vi "main.vi"() -> ()   [LabVIEW 2023] (continued)
C4\r\n      3444  0CF102A7   00000004    8        30\t75\tE0\t2E\t80\tFF\tFF\tFD\r\n      3443  0C3C4D4A   00000004    8        BE\tFF\tFF\t7F\t18\tFF\tFF\t5A\r\n      3443  0CF101A7   00000004    8        68\t00\t97\tCC\t00\t19\t39\tC6\r\n      3442  18F120F0   00000004    8        2B\t75\t60\tB1\tB0\t01\tFF\tFF\r\n      3441  18F11FF0   00000004    8        FF\t3F\t90\t68\t88\t1B\t10\tAC\r\n      3432  1FFFFFFF   00000004    8        00\t00\tFF\tFF\tFF\tFF\tFF\tFF\r\n      3423  0CF102A7   00000004    8        30\t75\tE0\t2E\t80\tFF\tFF\tFD\r\n      3423  0CF101A7   00000004    8        68\t00\t97\tCC\t00\t19\t39\tC5\r\n      3422  1FFFFFFF   00000004    8        00\t00\tFF\tFF\tFF\tFF\tFF\tFF\r\n      3412  1FFFFFFF   00000004    8        00\t00\tFF\tFF\tFF\tFF\tFF\tFF\r\n      3403  0CF102A7   00000004    8        30\t75\tE0\t2E\t80\tFF\tFF\tFD\r\n      3444  0CF103A7   00000004    8        17\t1F\t08\t60\tB1\t1F\t08\t5A\r\n      3444  0CF102A7   00000004    8        30\t75\tE0\t2E\t80\tFF\tFF\tFD\r\n      3443  0C3C4D4A   00000004    8        BE\tFF\tFF\t7F\t18\tFF\tFF\t5A\r\n      3443  0CF101A7   00000004    8        68\t00\t97\tCC\t00\t19\t39\tC6\r\n      3442  18F120F0   00000004    8        2B\t75\t60\tB1\tB0\t01\tFF\tFF\r\n      3441  18F11FF0   00000004    8        FF\t3F\t90\t68\t88\t1B\t10\tAC\r\n      3432  1FFFFFFF   00000004    8        00\t00\tFF\tFF\tFF\tFF\tFF\tFF\r\n      3423  0CF102A7   00000004    8        30\t75\tE0\t2E\t80\tFF\tFF\tFD\r\n      3423  0CF101A7   00000004    8        68\t00\t97\tCC\t00\t19\t39\tC5\r\n      3422  1FFFFFFF   00000004    8        00\t00\tFF\tFF\tFF\tFF\tFF\tFF\r\n      3412  1FFFFFFF   00000004    8        00\t00\tFF\tFF\tFF\tFF\tFF\tFF\r\n      3445  0CF104A7   00000004    8        F0\t60\t22\tFC\tFF\tFF\tFF\t5A\r\n      3444  0CF103A7   00000004    8        17\t1F\t08\t60\tB1\t1F\t08\t5A\r\n      3444  0CF102A7   00000004    8        30\t75\tE0\t2E\t80\tFF\tFF\tFD\r\n      3443  0C3C4D4A   00000004    8        BE\tFF\tFF\t7F\t18\tFF\tFF\t5A\r\n      3443  0CF101A7   00000004    8        68\t00\t97\tCC\t00\t19\t39\tC6\r\n      3442  18F120F0   00000004    8        2B\t75\t60\tB1\tB0\t01\tFF\tFF\r\n      3441  18F11FF0   00000004    8        FF\t3F\t90\t68\t88\t1B\t10\tAC\r\n      3432  1FFFFFFF   00000004    8        00\t00\tFF\tFF\tFF\tFF\tFF\tFF\r\n      3423  0CF102A7   00000004    8        30\t75\tE0\t2E\t80\tFF\tFF\tFD\r\n      3423  0CF101A7   00000004    8        68\t00\t97\tCC\t00\t19\t39\tC5\r\n      3422  1FFFFFFF   00000004    8        00\t00\tFF\tFF\tFF\tFF\tFF\tFF\r\n      3445  18F106A7   00000004    8        00\tF7\tFF\tFF\tFF\tFF\tFF\tB5\r\n      3445  0CF104A7   00000004    8        F0\t60\t22\tFC\tFF\tFF\tFF\t5A\r\n      3444  0CF103A7   00000004    8        17\t1F\t08\t60\tB1\t1F\t08\t5A\r\n      3444  0CF102A7   00000004    8        30\t75\tE0\t2E\t80\tFF\tFF\tFD\r\n      3443  0C3C4D4A   00000004    8        BE\tFF\tFF\t7F\t18\tFF\tFF\t5A\r\n      3443  0CF101A7   00000004    8        68\t00\t97\tCC\t00\t19\t39\tC6\r\n      3442  18F120F0   00000004    8        2B\t75\t60\tB1\tB0\t01\tFF\tFF\r\n      3441  18F11FF0   00000004    8        FF\t3F\t90\t68\t88\t1B\t10\tAC\r\n      3432  1FFFFFFF   00000004    8        00\t00\tFF\tFF\tFF\tFF\tFF\tFF\r\n      3423  0CF102A7   00000004    8        30\t75\tE0\t2E\t80\tFF\tFF\tFD\r\n      3423  0CF101A7   00000004    8        68\t00\t97\tCC\t00\t19\t39\tC5\r\n      3446  18F121F0   00000004    8        09\t33\t00\t00\tFF\tFF\tB0\t01\r\n      3445  18F106A7   00000004    8        00\tF7\tFF\tFF\tFF\tFF\tFF\tB5\r\n      3445  0CF104A7   00000004    8        F0\t60\t22\tFC\tFF\tFF\tFF\t5A\r\n      3444  0CF103A7   00000004    8        17\t1F\t08\t60\tB1\t1F\t08\t5A\r\n      3444  0CF102A7   00000004    8        30\t75\tE0\t2E\t80\tFF\tFF\tFD\r\n      3443  0C3C4D4A   00000004    8        BE\tFF\tFF\t7F\t18\tFF\tFF\t5A\r\n      3443  0CF101A7   00000004    8        68\t00\t97\tCC\t00\t19\t39\tC6\r\n      3442  18F120F0   00000004    8        2B\t75\t60\tB1\tB0\t01\tFF\tFF\r\n      3441  18F11FF0   00000004    8        FF\t3F\t90\t68\t88\t1B\t10\tAC\r\n      3432  1FFFFFFF   00000004    8        00\t00\tFF\tFF\tFF\tFF\tFF\tFF\r\n      3423  0CF102A7   00000004    8        30\t75\tE0\t2E\t80\tFF\tFF\tFD\r\n      3447  1FFFFFFF   00000004    8        00\t00\tFF\tFF\tFF\tFF\tFF\tFF\r\n      3446  18F121F0   00000004    8        09\t33\t00\t00\tFF\tFF\tB0\t01\r\n      3445  18F106A7   00000004    8        00\tF7\tFF\tFF\tFF\tFF\tFF\tB5\r\n      3445  0CF104A7   00000004    8        F0\t60\t22\tFC\tFF\tFF\tFF\t5A\r\n      3444  0CF103A7   00000004    8        17\t1F\t08\t60\tB1\t1F\t08\t5A\r\n      3444  0CF102A7   00000004    8        30\t75\tE0\t2E\t80\tFF\tFF\tFD\r\n      3443  0C3C4D4A   00000004    8        BE\tFF\tFF\t7F\t18\tFF\tFF\t5A\r\n      3443  0CF101A7   00000004    8        68\t00\t97\tCC\t00\t19\t39\tC6\r\n      3442  18F120F0   00000004    8        2B\t75\t60\tB1\tB0\t01\tFF\tFF\r\n      3441  18F11FF0   00000004    8        FF\t3F\t90\t68\t88\t1B\t10\tAC\r\n      3432  1FFFFFFF   00000004    8        00\t00\tFF\tFF\tFF\tFF\tFF\tFF\r\n      3452  1FFFFFFF   00000004    8        00\t00\tFF\tFF\tFF\tFF\tFF\tFF\r\n      3447  1FFFFFFF   00000004    8        00\t00\tFF\tFF\tFF\tFF\tFF\tFF\r\n      3446  18F121F0   00000004    8        09\t33\t00\t00\tFF\tFF\tB0\t01\r\n      3445  18F106A7   00000004    8        00\tF7\tFF\tFF\tFF\tFF\tFF\tB5\r\n      3445  0CF104A7   00000004    8        F0\t60\t22\tFC\tFF\tFF\tFF\t5A\r\n      3444  0CF103A7   00000004    8        17\t1F\t08\t60\tB1\t1F\t08\t5A\r\n      3444  0CF102A7   00000004    8        30\t75\tE0\t2E\t80\tFF\tFF\tFD\r\n      3443  0C3C4D4A   00000004    8        BE\tFF\tFF\t7F\t18\tFF\tFF\t5A\r\n      3443  0CF101A7   00000004    8        68\t00\t97\tCC\t00\t19\t39\tC6\r\n      3442  18F120F0   00000004    8        2B\t75\t60\tB1\tB0\t01\tFF\tFF\r\n      3441  18F11FF0   00000004    8        FF\t3F\t90\t68\t88\t1B\t10\tAC\r\n      3462  1FFFFFFF   00000004    8        00\t20\tFF\tFF\tFF\tFF\tFF\tFF\r\n      3452  1FFFFFFF   00000004    8        00\t00\tFF\tFF\tFF\tFF\tFF\tFF\r\n      3447  1FFFFFFF   00000004    8        00\t00\tFF\tFF\tFF\tFF\tFF\tFF\r\n      3446  18F121F0   00000004    8        09\t33\t00\t00\tFF\tFF\tB0\t01\r\n      3445  18F106A7   00000004    8        00\tF7\tFF\tFF\tFF\tFF\tFF\tB5\r\n      3445  0CF104A7   00000004    8        F0\t60\t22\tFC\tFF\tFF\tFF\t5A\r\n      3444  0CF103A7   00000004    8        17\t1F\t08\t60\tB1\t1F\t08\t5A\r\n      3444  0CF102A7   00000004    8        30\t75\tE0\t2E\t80\tFF\tFF\tFD\r\n      3443  0C3C4D4A   00000004    8        BE\tFF\tFF\t7F\t18\tFF\tFF\t5A\r\n      3443  0CF101A7   00000004    8        68\t00\t97\tCC\t00\t19\t39\tC6\r\n      3442  18F120F0   00000004    8        2B\t75\t60\tB1\tB0\t01\tFF\tFF\r\n      3463  0CF101A7   00000004    8        68\t00\t97\tCC\t00\t19\t39\tC7\r\n      3462  1FFFFFFF   00000004    8        00\t20\tFF\tFF\tFF\tFF\tFF\tFF\r\n      3452  1FFFFFFF   00000004    8        00\t00\tFF\tFF\tFF\tFF\tFF\tFF\r\n      3447  1FFFFFFF   00000004    8        00\t00\tFF\tFF\tFF\tFF\tFF\tFF\r\n      3446  18F121F0   00000004    8        09\t33\t00\t00\tFF\tFF\tB0\t01\r\n      3445  18F106A7   00000004    8        00\tF7\tFF\tFF\tFF\tFF\tFF\tB5\r\n      3445  0CF104A7   00000004    8        F0\t60\t22\tFC\tFF\tFF\tFF\t5A\r\n      3444  0CF103A7   00000004    8        17\t1F\t08\t60\tB1\t1F\t08\t5A\r\n      3444  0CF102A7   00000004    8        30\t75\tE0\t2E\t80\tFF\tFF\tFD\r\n      3443  0C3C4D4A   00000004    8        BE\tFF\tFF\t7F\t18\tFF\tFF\t5A\r\n      3443  0CF101A7   00000004    8        68\t00\t97\tCC\t00\t19\t39\tC6\r\n      3463  0CF102A7   00000004    8        30\t75\tE0\t2E\t80\tFF\tFF\tFD\r\n      3463  0CF101A7   00000004    8        68\t00\t97\tCC\t00\t19\t39\tC7\r\n      3462  1FFFFFFF   00000004    8        00\t20\tFF\tFF\tFF\tFF\tFF\tFF\r\n      3452  1FFFFFFF   00000004    8        00\t00\tFF\tFF\tFF\tFF\tFF\tFF\r\n      3447  1FFFFFFF   00000004    8        00\t00\tFF\tFF\tFF\tFF\tFF\tFF\r\n      3446  18F121F0   00000004    8        09\t33\t00\t00\tFF\tFF\tB0\t01\r\n      3445  18F106A7   00000004    8        00\tF7\tFF\tFF\tFF\tFF\tFF\tB5\r\n      3445  0CF104A7   00000004    8        F0\t60\t22\tFC\tFF\tFF\tFF\t5A\r\n      3444  0CF103A7   00000004    8        17\t1F\t08\t60\tB1\t1F\t08\t5A\r\n      3444  0CF102A7   00000004    8        30\t75\tE0\t2E\t80\tFF\tFF\tFD\r\n      3443  0C3C4D4A   00000004    8        BE\tFF\tFF\t7F\t18\tFF\tFF\t5A\r\n      3472  1FFFFFFF   00000004    8        00\t20\tFF\tFF\tFF\tFF\tFF\tFF\r\n      3463  0CF102A7   00000004    8        30\t75\tE0\t2E\t80\tFF\tFF\tFD\r\n      3463  0CF101A7   00000004    8        68\t00\t97\tCC\t00\t19\t39\tC7\r\n      3462  1FFFFFFF   00000004    8        00\t20\tFF\tFF\tFF\tFF\tFF\tFF\r\n      3452  1FFFFFFF   00000004    8        00\t00\tFF\tFF\tFF\tFF\tFF\tFF\r\n      3447  1FFFFFFF   00000004    8        00\t00\tFF\tFF\tFF\tFF\tFF\tFF\r\n      3446  18F121F0   00000004    8        09\t33\t00\t00\tFF\tFF\tB0\t01\r\n      3445  18F106A7   00000004    8        00\tF7\tFF\tFF\tFF\tFF\tFF\tB5\r\n      3445  0CF104A7   00000004    8        F0\t60\t22\tFC\tFF\tFF\tFF\t5A\r\n      3444  0CF103A7   00000004    8        17\t1F\t08\t60\tB1\t1F\t08\t5A\r\n      3444  0CF102A7   00000004    8        30\t75\tE0\t2E\t80\tFF\tFF\tFD\r\n      3482  1FFFFFFF   00000004    8        00\t20\tFF\tFF\tFF\tFF\tFF\tFF\r\n      3472  1FFFFFFF   00000004    8        00\t20\tFF\tFF\tFF\tFF\tFF\tFF\r\n      3463  0CF102A7   00000004    8        30\t75\tE0\t2E\t80\tFF\tFF\tFD\r\n      3463  0CF101A7   00000004    8        68\t00\t97\tCC\t00\t19\t39\tC7\r\n      3462  1FFFFFFF   00000004    8        00\t20\tFF\tFF\tFF\tFF\tFF\tFF\r\n      3452  1FFFFFFF   00000004    8        00\t00\tFF\tFF\tFF\tFF\tFF\tFF\r\n      3447  1FFFFFFF   00000004    8        00\t00\tFF\tFF\tFF\tFF\tFF\tFF\r\n      3446  18F121F0   00000004    8        09\t33\t00\t00\tFF\tFF\tB0\t01\r\n      3445  18F106A7   00000004    8        00\tF7\tFF\tFF\tFF\tFF\tFF\tB5\r\n      3445  0CF104A7   00000004    8        F0\t60\t22\tFC\tFF\tFF\tFF\t5A\r\n      3444  0CF103A7   00000004    8        17\t1F\t08\t60\tB1\t1F\t08\t5A\r\n      3483  0CF101A7   00000004    8        68\t00\t97\tCC\t00\t19\t39\tC8\r\n      3482  1FFFFFFF   00000004    8        00\t20\tFF\tFF\tFF\tFF\tFF\tFF\r\n      3472  1FFFFFFF   00000004    8        00\t20\tFF\tFF\tFF\tFF\tFF\tFF\r\n      3463  0CF102A7   00000004    8        30\t75\tE0\t2E\t80\tFF\tFF\tFD\r\n      3463  0CF101A7   00000004    8        68\t00\t97\tCC\t00\t19\t39\tC7\r\n      3462  1FFFFFFF   00000004    8        00\t20\tFF\tFF\tFF\tFF\tFF\tFF\r\n      3452  1FFFFFFF   00000004    8        00\t00\tFF\tFF\tFF\tFF\tFF\tFF\r\n      3447  1FFFFFFF   00000004    8        00\t00\tFF\tFF\tFF\tFF\tFF\tFF\r\n      3446  18F121F0   00000004    8        09\t33\t00\t00\tFF\tFF\tB0\t01\r\n      3445  18F106A7   00000004    8        00\tF7\tFF\tFF\tFF\tFF\tFF\tB5\r\n      3445  0CF104A7   00000004    8        F0\t60\t22\tFC\tFF\tFF\tFF\t5A\r\n      3483  0CF102A7   00000004    8        30\t75\tE0\t2E\t80\tFF\tFF\tFD\r\n      3483  0CF101A7   00000004    8        68\t00\t97\tCC\t00\t19\t39\tC8\r\n      3482  1FFFFFFF   00000004    8        00\t20\tFF\tFF\tFF\tFF\tFF\tFF\r\n      3472  1FFFFFFF   00000004    8        00\t20\tFF\tFF\tFF\tFF\tFF\tFF\r\n      3463  0CF102A7   00000004    8        30\t75\tE0\t2E\t80\tFF\tFF\tFD\r\n      3463  0CF101A7   00000004    8        68\t00\t97\tCC\t00\t19\t39\tC7\r\n      3462  1FFFFFFF   00000004    8        00\t20\tFF\tFF\tFF\tFF\tFF\tFF\r\n      3452  1FFFFFFF   00000004    8        00\t00\tFF\tFF\tFF\tFF\tFF\tFF\r\n      3447  1FFFFFFF   00000004    8        00\t00\tFF\tFF\tFF\tFF\tFF\tFF\r\n      3446  18F121F0   00000004    8        09\t33\t00\t00\tFF\tFF\tB0\t01\r\n      3445  18F106A7   00000004    8        00\tF7\tFF\tFF\tFF\tFF\tFF\tB5\r\n      3492  1FFFFFFF   00000004    8        00\t00\tFF\tFF\tFF\tFF\tFF\tFF\r\n      3483  0CF102A7   00000004    8        30\t75\tE0\t2E\t80\tFF\tFF\tFD\r\n      3483  0CF101A7   00000004    8        68\t00\t97\tCC\t00\t19\t39\tC8\r\n      3482  1FFFFFFF   00000004    8        00\t20\tFF\tFF\tFF\tFF\tFF\tFF\r\n      3472  1FFFFFFF   00000004    8        00\t20\tFF\tFF\tFF\tFF\tFF\tFF\r\n      3463  0CF102A7   00000004    8        30\t75\tE0\t2E\t80\tFF\tFF\tFD\r\n      3463  0CF101A7   00000004    8        68\t00\t97\tCC\t00\t19\t39\tC7\r\n      3462  1FFFFFFF   00000004    8        00\t20\tFF\tFF\tFF\tFF\tFF\tFF\r\n      3452  1FFFFFFF   00000004    8        00\t00\tFF\tFF\tFF\tFF\tFF\tFF\r\n      3447  1FFFFFFF   00000004    8        00\t00\tFF\tFF\tFF\tFF\tFF\tFF\r\n      3446  18F121F0   00000004    8        09\t33\t00\t00\tFF\tFF\tB0\t01\r\n      3493  18F106A7   00000004    8        00\tF7\tFF\tFF\tFF\tFF\tFF\tB6\r\n      3492  1FFFFFFF   00000004    8        00\t00\tFF\tFF\tFF\tFF\tFF\tFF\r\n      3483  0CF102A7   00000004    8        30\t75\tE0\t2E\t80\tFF\tFF\tFD\r\n      3483  0CF101A7   00000004    8        68\t00\t97\tCC\t00\t19\t39\tC8\r\n      3482  1FFFFFFF   00000004    8        00\t20\tFF\tFF\tFF\tFF\tFF\tFF\r\n      3472  1FFFFFFF   00000004    8        00\t20\tFF\tFF\tFF\tFF\tFF\tFF\r\n      3463  0CF102A7   00000004    8        30\t75\tE0\t2E\t80\tFF\tFF\tFD\r\n      3463  0CF101A7   00000004    8        68\t00\t97\tCC\t00\t19\t39\tC7\r\n      3462  1FFFFFFF   00000004    8        00\t20\tFF\tFF\tFF\tFF\tFF\tFF\r\n      3452  1FFFFFFF   00000004    8        00\t00\tFF\tFF\tFF\tFF\tFF\tFF\r\n      3447  1FFFFFFF   00000004    8        00\t00\tFF\tFF\tFF\tFF\tFF\tFF\r\n      3502  1FFFFFFF   00000004    8        00\t20\tFF\tFF\tFF\tFF\tFF\tFF\r\n      3493  18F106A7   00000004    8        00\tF7\tFF\tFF\tFF\tFF\tFF\tB6\r\n      3492  1FFFFFFF   00000004    8        00\t00\tFF\tFF\tFF\tFF\tFF\tFF\r\n      3483  0CF102A7   00000004    8        30\t75\tE0\t2E\t80\tFF\tFF\tFD\r\n      3483  0CF101A7   00000004    8        68\t00\t97\tCC\t00\t19\t39\tC8\r\n      3482  1FFFFFFF   00000004    8        00\t20\tFF\tFF\tFF\tFF\tFF\tFF\r\n      3472  1FFFFFFF   00000004    8        00\t20\tFF\tFF\tFF\tFF\tFF\tFF\r\n      3463  0CF102A7   00000004    8        30\t75\tE0\t2E\t80\tFF\tFF\tFD\r\n      3463  0CF101A7   00000004    8        68\t00\t97\tCC\t00\t19\t39\tC7\r\n      3462  1FFFFFFF   00000004    8        00\t20\tFF\tFF\tFF\tFF\tFF\tFF\r\n      3452  1FFFFFFF   00000004    8        00\t00\tFF\tFF\tFF\tFF\tFF\tFF\r\n      3503  0CF101A7   00000004    8        68\t00\t97\tCC\t00\t19\t39\tC9\r\n      3502  1FFFFFFF   00000004    8        00\t20\tFF\tFF\tFF\tFF\tFF\tFF\r\n      3493  18F106A7   00000004    8        00\tF7\tFF\tFF\tFF\tFF\tFF\tB6\r\n      3492  1FFFFFFF   00000004    8        00\t00\tFF\tFF\tFF\tFF\tFF\tFF\r\n      3483  0CF102A7   00000004    8        30\t75\tE0\t2E\t80\tFF\tFF\tFD\r\n      3483  0CF101A7   00000004    8        68\t00\t97\tCC\t00\t19\t39\tC8\r\n      3482  1FFFFFFF   00000004    8        00\t20\tFF\tFF\tFF\tFF\tFF\tFF\r\n      3472  1FFFFFFF   00000004    8        00\t20\tFF\tFF\tFF\tFF\tFF\tFF\r\n      3463  0CF102A7   00000004    8        30\t75\tE0\t2E\t80\tFF\tFF\tFD\r\n      3463  0CF101A7   00000004    8        68\t00\t97\tCC\t00\t19\t39\tC7\r\n      3462  1FFFFFFF   00000004    8        00\t20\tFF\tFF\tFF\tFF\tFF\tFF\r\n      3503  0CF102A7   00000004    8        30\t75\tE0\t2E\t80\tFF\tFF\tFD\r\n      3503  0CF101A7   00000004    8        68\t00\t97\tCC\t00\t19\t39\tC9\r\n      3502  1FFFFFFF   00000004    8        00\t20\tFF\tFF\tFF\tFF\tFF\tFF\r\n      3493  18F106A7   00000004    8        00\tF7\tFF\tFF\tFF\tFF\tFF\tB6\r\n      3492  1FFFFFFF   00000004    8        00\t00\tFF\tFF\tFF\tFF\tFF\tFF\r\n      3483  0CF102A7   00000004    8        30\t75\tE0\t2E\t80\tFF\tFF\tFD\r\n      3483  0CF101A7   00000004    8        68\t00\t97\tCC\t00\t19\t39\tC8\r\n      3482  1FFFFFFF   00000004    8        00\t20\tFF\tFF\tFF\tFF\tFF\tFF\r\n      3472  1FFFFFFF   00000004    8        00\t20\tFF\tFF\tFF\tFF\tFF\tFF\r\n      3463  0CF102A7   00000004    8        30\t75\tE0\t2E\t80\tFF\tFF\tFD\r\n      3463  0CF101A7   00000004    8        68\t00\t97\tCC\t00\t19\t39\tC7\r\n      3512  1FFFFFFF   00000004    8        00\t20\tFF\tFF\tFF\tFF\tFF\tFF\r\n      3503  0CF102A7   00000004    8        30\t75\tE0\t2E\t80\tFF\tFF\tFD\r\n      3503  0CF101A7   00000004    8        68\t00\t97\tCC\t00\t19\t39\tC9\r\n      3502  1FFFFFFF   00000004    8        00\t20\tFF\tFF\tFF\tFF\tFF\tFF\r\n      3493  18F106A7   00000004    8        00\tF7\tFF\tFF\tFF\tFF\tFF\tB6\r\n      3492  1FFFFFFF   00000004    8        00\t00\tFF\tFF\tFF\tFF\tFF\tFF\r\n      3483  0CF102A7   00000004    8        30\t75\tE0\t2E\t80\tFF\tFF\tFD\r\n      3483  0CF101A7   00000004    8        68\t00\t97\tCC\t00\t19\t39\tC8\r\n      3482  1FFFFFFF   00000004    8        00\t20\tFF\tFF\tFF\tFF\tFF\tFF\r\n      3472  1FFFFFFF   00000004    8        00\t20\tFF\tFF\tFF\tFF\tFF\tFF\r\n      3463  0CF102A7   00000004    8        30\t75\tE0\t2E\t80\tFF\tFF\tFD\r\n      3522  1FFFFFFF   00000004    8        00\t00\tFF\tFF\tFF\tFF\tFF\tFF\r\n      3512  1FFFFFFF   00000004    8        00\t20\tFF\tFF\tFF\tFF\tFF\tFF\r\n      3503  0CF102A7   00000004    8        30\t75\tE0\t2E\t80\tFF\tFF\tFD\r\n      3503  0CF101A7   00000004    8        68\t00\t97\tCC\t00\t19\t39\tC9\r\n      3502  1FFFFFFF   00000004    8        00\t20\tFF\tFF\tFF\tFF\tFF\tFF\r\n      3493  18F106A7   00000004    8        00\tF7\tFF\tFF\tFF\tFF\tFF\tB6\r\n      3492  1FFFFFFF   00000004    8        00\t00\tFF\tFF\tFF\tFF\tFF\tFF\r\n      3483  0CF102A7   00000004    8        30\t75\tE0\t2E\t80\tFF\tFF\tFD\r\n      3483  0CF101A7   00000004    8        68\t00\t97\tCC\t00\t19\t39\tC8\r\n      3482  1FFFFFFF   00000004    8        00\t20\tFF\tFF\tFF\tFF\tFF\tFF\r\n      3472  1FFFFFFF   00000004    8        00\t20\tFF\tFF\tFF\tFF\tFF\tFF\r\n      3523  0CF101A7   00000004    8        68\t00\t97\tCC\t00\t19\t39\tCA\r\n      3522  1FFFFFFF   00000004    8        00\t00\tFF\tFF\tFF\tFF\tFF\tFF\r\n      3512  1FFFFFFF   00000004    8        00\t20\tFF\tFF\tFF\tFF\tFF\tFF\r\n      3503  0CF102A7   00000004    8        30\t75\tE0\t2E\t80\tFF\tFF\tFD\r\n      3503  0CF101A7   00000004    8        68\t00\t97\tCC\t00\t19\t39\tC9\r\n      3502  1FFFFFFF   00000004    8        00\t20\tFF\tFF\tFF\tFF\tFF\tFF\r\n      3493  18F106A7   00000004    8        00\tF7\tFF\tFF\tFF\tFF\tFF\tB6\r\n      3492  1FFFFFFF   00000004    8        00\t00\tFF\tFF\tFF\tFF\tFF\tFF\r\n      3483  0CF102A7   00000004    8        30\t75\tE0\t2E\t80\tFF\tFF\tFD\r\n      3483  0CF101A7   00000004    8        68\t00\t97\tCC\t00\t19\t39\tC8\r\n      3482  1FFFFFFF   00000004    8        00\t20\tFF\tFF\tFF\tFF\tFF\tFF\r\n      3523  0CF102A7   00000004    8        30\t75\tE0\t2E\t80\tFF\tFF\tFD\r\n      3523  0CF101A7   00000004    8        68\t00\t97\tCC\t00\t19\t39\tCA\r\n      3522  1FFFFFFF   00000004    8        00\t00\tFF\tFF\tFF\tFF\tFF\tFF\r\n      3512  1FFFFFFF   00000004    8        00\t20\tFF\tFF\tFF\tFF\tFF\tFF\r\n      3503  0CF102A7   00000004    8        30\t75\tE0\t2E\t80\tFF\tFF\tFD\r\n      3503  0CF101A7   00000004    8        68\t00\t97\tCC\t00\t19\t39\tC9\r\n      3502  1FFFFFFF   00000004    8        00\t20\tFF\tFF\tFF\tFF\tFF\tFF\r\n      3493  18F106A7   00000004    8        00\tF7\tFF\tFF\tFF\tFF\tFF\tB6\r\n      3492  1FFFFFFF   00000004    8        00\t00\tFF\tFF\tFF\tFF\tFF\tFF\r\n      3483  0CF102A7   00000004    8        30\t75\tE0\t2E\t80\tFF\tFF\tFD\r\n      3483  0CF101A7   00000004    8        68\t00\t97\tCC\t00\t19\t39\tC8\r\n      3532  1FFFFFFF   00000004    8        00\t20\tFF\tFF\tFF\tFF\tFF\tFF\r\n      3523  0CF102A7   00000004    8        30\t75\tE0\t2E\t80\tFF\tFF\tFD\r\n      3523  0CF101A7   00000004    8        68\t00\t97\tCC\t00\t19\t39\tCA\r\n      3522  1FFFFFFF   00000004    8        00\t00\tFF\tFF\tFF\tFF\tFF\tFF\r\n      3512  1FFFFFFF   00000004    8        00\t20\tFF\tFF\tFF\tFF\tFF\tFF\r\n      3503  0CF102A7   00000004    8        30\t75\tE0\t2E\t80\tFF\tFF\tFD\r\n      3503  0CF101A7   00000004    8        68\t00\t97\tCC\t00\t19\t39\tC9\r\n      3502  1FFFFFFF   00000004    8        00\t20\tFF\tFF\tFF\tFF\tFF\tFF\r\n      3493  18F106A7   00000004    8        00\tF7\tFF\tFF\tFF\tFF\tFF\tB6\r\n      3492  1FFFFFFF   00000004    8        00\t00\tFF\tFF\tFF\tFF\tFF\tFF\r\n      3483  0CF102A7   00000004    8        30\t75\tE0\t2E\t80\tFF\tFF\tFD\r\n      3541  18F11FF0   00000004    8        FF\t3F\t90\t68\t88\t1B\t10\tBC\r\n      3532  1FFFFFFF   00000004    8        00\t20\tFF\tFF\tFF\tFF\tFF\tFF\r\n      3523  0CF102A7   00000004    8        30\t75\tE0\t2E\t80\tFF\tFF\tFD\r\n      3523  0CF101A7   00000004    8        68\t00\t97\tCC\t00\t19\t39\tCA\r\n      3522  1FFFFFFF   00000004    8        00\t00\tFF\tFF\tFF\tFF\tFF\tFF\r\n      3512  1FFFFFFF   00000004    8        00\t20\tFF\tFF\tFF\tFF\tFF\tFF\r\n      3503  0CF102A7   00000004    8        30\t75\tE0\t2E\t80\tFF\tFF\tFD\r\n      3503  0CF101A7   00000004    8        68\t00\t97\tCC\t00\t19\t39\tC9\r\n      3502  1FFFFFFF   00000004    8        00\t20\tFF\tFF\tFF\tFF\tFF\tFF\r\n      3493  18F106A7   00000004    8        00\tF7\tFF\tFF\tFF\tFF\tFF\tB6\r\n      3492  1FFFFFFF   00000004    8        00\t00\tFF\tFF\tFF\tFF\tFF\tFF\r\n      3542  18F120F0   00000004    8        2B\t75\t60\tB1\tB0\t01\tFF\tFF\r\n      3541  18F11FF0   00000004    8        FF\t3F\t90\t68\t88\t1B\t10\tBC\r\n      3532  1FFFFFFF   00000004    8        00\t20\tFF\tFF\tFF\tFF\tFF\tFF\r\n      3523  0CF102A7   00000004    8        30\t75\tE0\t2E\t80\tFF\tFF\tFD\r\n      3523  0CF101A7   00000004    8        68\t00\t97\tCC\t00\t19\t39\tCA\r\n      3522  1FFFFFFF   00000004    8        00\t00\tFF\tFF\tFF\tFF\tFF\tFF\r\n      3512  1FFFFFFF   00000004    8        00\t20\tFF\tFF\tFF\tFF\tFF\tFF\r\n      3503  0CF102A7   00000004    8        30\t75\tE0\t2E\t80\tFF\tFF\tFD\r\n      3503  0CF101A7   00000004    8        68\t00\t97\tCC\t00\t19\t39\tC9\r\n      3502  1FFFFFFF   00000004    8        00\t20\tFF\tFF\tFF\tFF\tFF\tFF\r\n      3493  18F106A7   00000004    8        00\tF7\tFF\tFF\tFF\tFF\tFF\tB6\r\n      3543  0CF101A7   00000004    8        68\t00\t97\tCC\t00\t19\t39\tCB\r\n      3542  18F120F0   00000004    8        2B\t75\t60\tB1\tB0\t01\tFF\tFF\r\n      3541  18F11FF0   00000004    8        FF\t3F\t90\t68\t88\t1B\t10\tBC\r\n      3532  1FFFFFFF   00000004    8        00\t20\tFF\tFF\tFF\tFF\tFF\tFF\r\n      3523  0CF102A7   00000004    8        30\t75\tE0\t2E\t80\tFF\tFF\tFD\r\n      3523  0CF101A7   00000004    8        68\t00\t97\tCC\t00\t19\t39\tCA\r\n      3522  1FFFFFFF   00000004    8        00\t00\tFF\tFF\tFF\tFF\tFF\tFF\r\n      3512  1FFFFFFF   00000004    8        00\t20\tFF\tFF\tFF\tFF\tFF\tFF\r\n      3503  0CF102A7   00000004    8        30\t75\tE0\t2E\t80\tFF\tFF\tFD\r\n      3503  0CF101A7   00000004    8        68\t00\t97\tCC\t00\t19\t39\tC9\r\n      3502  1FFFFFFF   00000004    8        00\t20\tFF\tFF\tFF\tFF\tFF\tFF\r\n      3543  0C3C4D4A   00000004    8        BE\tFF\tFF\t7F\t18\tFF\tFF\t5B\r\n      3543  0CF101A7   00000004    8        68\t00\t97\tCC\t00\t19\t39\tCB\r\n      3542  18F120F0   00000004    8        2B\t75\t60\tB1\tB0\t01\tFF\tFF\r\n      3541  18F11FF0   00000004    8        FF\t3F\t90\t68\t88\t1B\t10\tBC\r\n      3532  1FFFFFFF   00000004    8        00\t20\tFF\tFF\tFF\tFF\tFF\tFF\r\n      3523  0CF102A7   00000004    8        30\t75\tE0\t2E\t80\tFF\tFF\tFD\r\n      3523  0CF101A7   00000004    8        68\t00\t97\tCC\t00\t19\t39\tCA\r\n      3522  1FFFFFFF   00000004    8        00\t00\tFF\tFF\tFF\tFF\tFF\tFF\r\n      3512  1FFFFFFF   00000004    8        00\t20\tFF\tFF\tFF\tFF\tFF\tFF\r\n      3503  0CF102A7   00000004    8        30\t75\tE0\t2E\t80\tFF\tFF\tFD\r\n      3503  0CF101A7   00000004    8        68\t00\t97\tCC\t00\t19\t39\tC9\r\n      3544  0CF102A7   00000004    8        30\t75\tE0\t2E\t80\tFF\tFF\tFD\r\n      3543  0C3C4D4A   00000004    8        BE\tFF\tFF\t7F\t18\tFF\tFF\t5B\r\n      3543  0CF101A7   00000004    8        68\t00\t97\tCC\t00\t19\t39\tCB\r\n      3542  18F120F0   00000004    8        2B\t75\t60\tB1\tB0\t01\tFF\tFF\r\n      3541  18F11FF0   00000004    8        FF\t3F\t90\t68\t88\t1B\t10\tBC\r\n      3532  1FFFFFFF   00000004    8        00\t20\tFF\tFF\tFF\tFF\tFF\tFF\r\n      3523  0CF102A7   00000004    8        30\t75\tE0\t2E\t80\tFF\tFF\tFD\r\n      3523  0CF101A7   00000004    8        68\t00\t97\tCC\t00\t19\t39\tCA\r\n      3522  1FFFFFFF   00000004    8        00\t00\tFF\tFF\tFF\tFF\tFF\tFF\r\n      3512  1FFFFFFF   00000004    8        00\t20\tFF\tFF\tFF\tFF\tFF\tFF\r\n      3503  0CF102A7   00000004    8        30\t75\tE0\t2E\t80\tFF\tFF\tFD\r\n      3544  0CF103A7   00000004    8        17\t1F\t08\t60\tB1\t1F\t08\t5B\r\n      3544  0CF102A7   00000004    8        30\t75\tE0\t2E\t80\tFF\tFF\tFD\r\n      3543  0C3C4D4A   00000004    8        BE\tFF\tFF\t7F\t18\tFF\tFF\t5B\r\n      3543  0CF101A7   00000004    8        68\t00\t97\tCC\t00\t19\t39\tCB\r\n      3542  18F120F0   00000004    8        2B\t75\t60\tB1\tB0\t01\tFF\tFF\r\n      3541  18F11FF0   00000004    8        FF\t3F\t90\t68\t88\t1B\t10\tBC\r\n      3532  1FFFFFFF   00000004    8        00\t20\tFF\tFF\tFF\tFF\tFF\tFF\r\n      3523  0CF102A7   00000004    8        30\t75\tE0\t2E\t80\tFF\tFF\tFD\r\n      3523  0CF101A7   00000004    8        68\t00\t97\tCC\t00\t19\t39\tCA\r\n      3522  1FFFFFFF   00000004    8        00\t00\tFF\tFF\tFF\tFF\tFF\tFF\r\n      3512  1FFFFFFF   00000004    8        00\t20\tFF\tFF\tFF\tFF\tFF\tFF\r\n      3545  0CF104A7   00000004    8        F0\t60\t22\tFC\tFF\tFF\tFF\t5B\r\n      3544  0CF103A7   00000004    8        17\t1F\t08\t60\tB1\t1F\t08\t5B\r\n      3544  0CF102A7   00000004    8        30\t75\tE0\t2E\t80\tFF\tFF\tFD\r\n      3543  0C3C4D4A   00000004    8        BE\tFF\tFF\t7F\t18\tFF\tFF\t5B\r\n      3543  0CF101A7   00000004    8        68\t00\t97\tCC\t00\t19\t39\tCB\r\n      3542  18F120F0   00000004    8        2B\t75\t60\tB1\tB0\t01\tFF\tFF\r\n      3541  18F11FF0   00000004    8        FF\t3F\t90\t68\t88\t1B\t10\tBC\r\n      3532  1FFFFFFF   00000004    8        00\t20\tFF\tFF\tFF\tFF\tFF\tFF\r\n      3523  0CF102A7   00000004    8        30\t75\tE0\t2E\t80\tFF\tFF\tFD\r\n      3523  0CF101A7   00000004    8        68\t00\t97\tCC\t00\t19\t39\tCA\r\n      3522  1FFFFFFF   00000004    8        00\t00\tFF\tFF\tFF\tFF\tFF\tFF\r\n      3545  18F106A7   00000004    8        00\tF7\tFF\tFF\tFF\tFF\tFF\tB7\r\n      3545  0CF104A7   00000004    8        F0\t60\t22\tFC\tFF\tFF\tFF\t5B\r\n      3544  0CF103A7   00000004    8        17\t1F\t08\t60\tB1\t1F\t08\t5B\r\n      3544  0CF102A7   00000004    8        30\t75\tE0\t2E\t80\tFF\tFF\tFD\r\n      3543  0C3C4D4A   00000004    8        BE\tFF\tFF\t7F\t18\tFF\tFF\t5B\r\n      3543  0CF101A7   00000004    8        68\t00\t97\tCC\t00\t19\t39\tCB\r\n      3542  18F120F0   00000004    8        2B\t75\t60\tB1\tB0\t01\tFF\tFF\r\n      3541  18F11FF0   00000004    8        FF\t3F\t90\t68\t88\t1B\t10\tBC\r\n      3532  1FFFFFFF   00000004    8        00\t20\tFF\tFF\tFF\tFF\tFF\tFF\r\n      3523  0CF102A7   00000004    8        30\t75\tE0\t2E\t80\tFF\tFF\tFD\r\n      3523  0CF101A7   00000004    8        68\t00\t97\tCC\t00\t19\t39\tCA\r\n      3546  18F121F0   00000004    8        09\t33\t00\t00\tFF\tFF\tB0\t01\r\n      3545  18F106A7   00000004    8        00\tF7\tFF\tFF\tFF\tFF\tFF\tB7\r\n      3545  0CF104A7   00000004    8        F0\t60\t22\tFC\tFF\tFF\tFF\t5B\r\n      3544  0CF103A7   00000004    8        17\t1F\t08\t60\tB1\t1F\t08\t5B\r\n      3544  0CF102A7   00000004    8        30\t75\tE0\t2E\t80\tFF\tFF\tFD\r\n      3543  0C3C4D4A   00000004    8        BE\tFF\tFF\t7F\t18\tFF\tFF\t5B\r\n      3543  0CF101A7   00000004    8        68\t00\t97\tCC\t00\t19\t39\tCB\r\n      3542  18F120F0   00000004    8        2B\t75\t60\tB1\tB0\t01\tFF\tFF\r\n      3541  18F11FF0   00000004    8        FF\t3F\t90\t68\t88\t1B\t10\tBC\r\n      3532  1FFFFFFF   00000004    8        00\t20\tFF\tFF\tFF\tFF\tFF\tFF\r\n      3523  0CF102A7   00000004    8        30\t75\tE0\t2E\t80\tFF\tFF\tFD\r\n      3547  1FFFFFFF   00000004    8        00\t00\tFF\tFF\tFF\tFF\tFF\tFF\r\n      3546  18F121F0   00000004    8        09\t33\t00\t00\tFF\tFF\tB0\t01\r\n      3545  18F106A7   00000004    8        00\tF7\tFF\tFF\tFF\tFF\tFF\tB7\r\n      3545  0CF104A7   00000004    8        F0\t60\t22\tFC\tFF\tFF\tFF\t5B\r\n      3544  0CF103A7   00000004    8        17\t1F\t08\t60\tB1\t1F\t08\t5B\r\n      3544  0CF102A7   00000004    8        30\t75\tE0\t2E\t80\tFF\tFF\tFD\r\n      3543  0C3C4D4A   00000004    8        BE\tFF\tFF\t7F\t18\tFF\tFF\t5B\r\n      3543  0CF101A7   00000004    8        68\t00\t97\tCC\t00\t19\t39\tCB\r\n      3542  18F120F0   00000004    8        2B\t75\t60\tB1\tB0\t01\tFF\tFF\r\n      3541  18F11FF0   00000004    8        FF\t3F\t90\t68\t88\t1B\t10\tBC\r\n      3532  1FFFFFFF   00000004    8        00\t20\tFF\tFF\tFF\tFF\tFF\tFF\r\n      3552  1FFFFFFF   00000004    8        00\t00\tFF\tFF\tFF\tFF\tFF\tFF\r\n      3547  1FFFFFFF   00000004    8        00\t00\tFF\tFF\tFF\tFF\tFF\tFF\r\n      3546  18F121F0   00000004    8        09\t33\t00\t00\tFF\tFF\tB0\t01\r\n      3545  18F106A7   00000004    8        00\tF7\tFF\tFF\tFF\tFF\tFF\tB7\r\n      3545  0CF104A7   00000004    8        F0\t60\t22\tFC\tFF\tFF\tFF\t5B\r\n      3544  0CF103A7   00000004    8        17\t1F\t08\t60\tB1\t1F\t08\t5B\r\n      3544  0CF102A7   00000004    8        30\t75\tE0\t2E\t80\tFF\tFF\tFD\r\n      3543  0C3C4D4A   00000004    8        BE\tFF\tFF\t7F\t18\tFF\tFF\t5B\r\n      3543  0CF101A7   00000004    8        68\t00\t97\tCC\t00\t19\t39\tCB\r\n      3542  18F120F0   00000004    8        2B\t75\t60\tB1\tB0\t01\tFF\tFF\r\n      3541  18F11FF0   00000004    8        FF\t3F\t90\t68\t88\t1B\t10\tBC\r\n      3562  1FFFFFFF   00000004    8        00\t20\tFF\tFF\tFF\tFF\tFF\tFF\r\n      3552  1FFFFFFF   00000004    8        00\t00\tFF\tFF\tFF\tFF\tFF\tFF\r\n      3547  1FFFFFFF   00000004    8        00\t00\tFF\tFF\tFF\tFF\tFF\tFF\r\n      3546  18F121F0   00000004    8        09\t33\t00\t00\tFF\tFF\tB0\t01\r\n      3545  18F106A7   00000004    8        00\tF7\tFF\tFF\tFF\tFF\tFF\tB7\r\n      3545  0CF104A7   00000004    8        F0\t60\t22\tFC\tFF\tFF\tFF\t5B\r\n      3544  0CF103A7   00000004    8        17\t1F\t08\t60\tB1\t1F\t08\t5B\r\n      3544  0CF102A7   00000004    8        30\t75\tE0\t2E\t80\tFF\tFF\tFD\r\n      3543  0C3C4D4A   00000004    8        BE\tFF\tFF\t7F\t18\tFF\tFF\t5B\r\n      3543  0CF101A7   00000004    8        68\t00\t97\tCC\t00\t19\t39\tCB\r\n      3542  18F120F0   00000004    8        2B\t75\t60\tB1\tB0\t01\tFF\tFF\r\n      3563  0CF101A7   00000004    8        68\t00\t97\tCC\t00\t19\t39\tCC\r\n      3562  1FFFFFFF   00000004    8        00\t20\tFF\tFF\tFF\tFF\tFF\tFF\r\n      3552  1FFFFFFF   00000004    8        00\t00\tFF\tFF\tFF\tFF\tFF\tFF\r\n      3547  1FFFFFFF   00000004    8        00\t00\tFF\tFF\tFF\tFF\tFF\tFF\r\n      3546  18F121F0   00000004    8        09\t33\t00\t00\tFF\tFF\tB0\t01\r\n      3545  18F106A7   00000004    8        00\tF7\tFF\tFF\tFF\tFF\tFF\tB7\r\n      3545  0CF104A7   00000004    8        F0\t60\t22\tFC\tFF\tFF\tFF\t5B\r\n      3544  0CF103A7   00000004    8        17\t1F\t08\t60\tB1\t1F\t08\t5B\r\n      3544  0CF102A7   00000004    8        30\t75\tE0\t2E\t80\tFF\tFF\tFD\r\n      3543  0C3C4D4A   00000004    8        BE\tFF\tFF\t7F\t18\tFF\tFF\t5B\r\n      3543  0CF101A7   00000004    8        68\t00\t97\tCC\t00\t19\t39\tCB\r\n      3563  0CF102A7   00000004    8        30\t75\tE0\t2E\t80\tFF\tFF\tFD\r\n      3563  0CF101A7   00000004    8        68\t00\t97\tCC\t00\t19\t39\tCC\r\n      3562  1FFFFFFF   00000004    8        00\t20\tFF\tFF\tFF\tFF\tFF\tFF\r\n      3552  1FFFFFFF   00000004    8        00\t00\tFF\tFF\tFF\tFF\tFF\tFF\r\n      3547  1FFFFFFF   00000004    8        00\t00\tFF\tFF\tFF\tFF\tFF\tFF\r\n      3546  18F121F0   00000004    8        09\t33\t00\t00\tFF\tFF\tB0\t01\r\n      3545  18F106A7   00000004    8        00\tF7\tFF\tFF\tFF\tFF\tFF\tB7\r\n      3545  0CF104A7   00000004    8        F0\t60\t22\tFC\tFF\tFF\tFF\t5B\r\n      3544  0CF103A7   00000004    8        17\t1F\t08\t60\tB1\t1F\t08\t5B\r\n      3544  0CF102A7   00000004    8        30\t75\tE0\t2E\t80\tFF\tFF\tFD\r\n      3543  0C3C4D4A   00000004    8        BE\tFF\tFF\t7F\t18\tFF\tFF\t5B\r\n      3572  1FFFFFFF   00000004    8        00\t20\tFF\tFF\tFF\tFF\tFF\tFF\r\n      3563  0CF102A7   00000004    8        30\t75\tE0\t2E\t80\tFF\tFF\tFD\r\n      3563  0CF101A7   00000004    8        68\t00\t97\tCC\t00\t19\t39\tCC\r\n      3562  1FFFFFFF   00000004    8        00\t20\tFF\tFF\tFF\tFF\tFF\tFF\r\n      3552  1FFFFFFF   00000004    8        00\t00\tFF\tFF\tFF\tFF\tFF\tFF\r\n      3547  1FFFFFFF   00000004    8        00\t00\tFF\tFF\tFF\tFF\tFF\tFF\r\n      3546  18F121F0   00000004    8        09\t33\t00\t00\tFF\tFF\tB0\t01\r\n      3545  18F106A7   00000004    8        00\tF7\tFF\tFF\tFF\tFF\tFF\tB7\r\n      3545  0CF104A7   00000004    8        F0\t60\t22\tFC\tFF\tFF\tFF\t5B\r\n      3544  0CF103A7   00000004    8        17\t1F\t08\t60\tB1\t1F\t08\t5B\r\n      3544  0CF102A7   00000004    8        30\t75\tE0\t2E\t80\tFF\tFF\tFD\r\n      3582  1FFFFFFF   00000004    8        00\t20\tFF\tFF\tFF\tFF\tFF\tFF\r\n      3572  1FFFFFFF   00000004    8        00\t20\tFF\tFF\tFF\tFF\tFF\tFF\r\n      3563  0CF102A7   00000004    8        30\t75\tE0\t2E\t80\tFF\tFF\tFD\r\n      3563  0CF101A7   00000004    8        68\t00\t97\tCC\t00\t19\t39\tCC\r\n      3562  1FFFFFFF   00000004    8        00\t20\tFF\tFF\tFF\tFF\tFF\tFF\r\n      3552  1FFFFFFF   00000004    8        00\t00\tFF\tFF\tFF\tFF\tFF\tFF\r\n      3547  1FFFFFFF   00000004    8        00\t00\tFF\tFF\tFF\tFF\tFF\tFF\r\n      3546  18F121F0   00000004    8        09\t33\t00\t00\tFF\tFF\tB0\t01\r\n      3545  18F106A7   00000004    8        00\tF7\tFF\tFF\tFF\tFF\tFF\tB7\r\n      3545  0CF104A7   00000004    8        F0\t60\t22\tFC\tFF\tFF\tFF\t5B\r\n      3544  0CF103A7   00000004    8        17\t1F\t08\t60\tB1\t1F\t08\t5B\r\n      3583  0CF101A7   00000004    8        68\t00\t97\tCC\t00\t19\t39\tCD\r\n      3582  1FFFFFFF   00000004    8        00\t20\tFF\tFF\tFF\tFF\tFF\tFF\r\n      3572  1FFFFFFF   00000004    8        00\t20\tFF\tFF\tFF\tFF\tFF\tFF\r\n      3563  0CF102A7   00000004    8        30\t75\tE0\t2E\t80\tFF\tFF\tFD\r\n      3563  0CF101A7   00000004    8        68\t00\t97\tCC\t00\t19\t39\tCC\r\n      3562  1FFFFFFF   00000004    8        00\t20\tFF\tFF\tFF\tFF\tFF\tFF\r\n      3552  1FFFFFFF   00000004    8        00\t00\tFF\tFF\tFF\tFF\tFF\tFF\r\n      3547  1FFFFFFF   00000004    8        00\t00\tFF\tFF\tFF\tFF\tFF\tFF\r\n      3546  18F121F0   00000004    8        09\t33\t00\t00\tFF\tFF\tB0\t01\r\n      3545  18F106A7   00000004    8        00\tF7\tFF\tFF\tFF\tFF\tFF\tB7\r\n      3545  0CF104A7   00000004    8        F0\t60\t22\tFC\tFF\tFF\tFF\t5B\r\n      3583  0CF102A7   00000004    8        30\t75\tE0\t2E\t80\tFF\tFF\tFD\r\n      3583  0CF101A7   00000004    8        68\t00\t97\tCC\t00\t19\t39\tCD\r\n      3582  1FFFFFFF   00000004    8        00\t20\tFF\tFF\tFF\tFF\tFF\tFF\r\n      3572  1FFFFFFF   00000004    8        00\t20\tFF\tFF\tFF\tFF\tFF\tFF\r\n      3563  0CF102A7   00000004    8        30\t75\tE0\t2E\t80\tFF\tFF\tFD\r\n      3563  0CF101A7   00000004    8        68\t00\t97\tCC\t00\t19\t39\tCC\r\n      3562  1FFFFFFF   00000004    8        00\t20\tFF\tFF\tFF\tFF\tFF\tFF\r\n      3552  1FFFFFFF   00000004    8        00\t00\tFF\tFF\tFF\tFF\tFF\tFF\r\n      3547  1FFFFFFF   00000004    8        00\t00\tFF\tFF\tFF\tFF\tFF\tFF\r\n      3546  18F121F0   00000004    8        09\t33\t00\t00\tFF\tFF\tB0\t01\r\n      3545  18F106A7   00000004    8        00\tF7\tFF\tFF\tFF\tFF\tFF\tB7\r\n      3592  1FFFFFFF   00000004    8        00\t00\tFF\tFF\tFF\tFF\tFF\tFF\r\n      3583  0CF102A7   00000004    8        30\t75\tE0\t2E\t80\tFF\tFF\tFD\r\n      3583  0CF101A7   00000004    8        68\t00\t97\tCC\t00\t19\t39\tCD\r\n      3582  1FFFFFFF   00000004    8        00\t20\tFF\tFF\tFF\tFF\tFF\tFF\r\n      3572  1FFFFFFF   00000004    8        00\t20\tFF\tFF\tFF\tFF\tFF\tFF\r\n      3563  0CF102A7   00000004    8        30\t75\tE0\t2E\t80\tFF\tFF\tFD\r\n      3563  0CF101A7   00000004    8        68\t00\t97\tCC\t00\t19\t39\tCC\r\n      3562  1FFFFFFF   00000004    8        00\t20\tFF\tFF\tFF\tFF\tFF\tFF\r\n      3552  1FFFFFFF   00000004    8        00\t00\tFF\tFF\tFF\tFF\tFF\tFF\r\n      3547  1FFFFFFF   00000004    8        00\t00\tFF\tFF\tFF\tFF\tFF\tFF\r\n      3546  18F121F0   00000004    8        09\t33\t00\t00\tFF\tFF\tB0\t01\r\n      3593  18F106A7   00000004    8        00\tF7\tFF\tFF\tFF\tFF\tFF\tB8\r\n      3592  1FFFFFFF   00000004    8        00\t00\tFF\tFF\tFF\tFF\tFF\tFF\r\n      3583  0CF102A7   00000004    8        30\t75\tE0\t2E\t80\tFF\tFF\tFD\r\n      3583  0CF101A7   00000004    8        68\t00\t97\tCC\t00\t19\t39\tCD\r\n      3582  1FFFFFFF   00000004    8        00\t20\tFF\tFF\tFF\tFF\tFF\tFF\r\n      3572  1FFFFFFF   00000004    8        00\t20\tFF\tFF\tFF\tFF\tFF\tFF\r\n      3563  0CF102A7   00000004    8        30\t75\tE0\t2E\t80\tFF\tFF\tFD\r\n      3563  0CF101A7   00000004    8        68\t00\t97\tCC\t00\t19\t39\tCC\r\n      3562  1FFFFFFF   00000004    8        00\t20\tFF\tFF\tFF\tFF\tFF\tFF\r\n      3552  1FFFFFFF   00000004    8        00\t00\tFF\tFF\tFF\tFF\tFF\tFF\r\n      3547  1FFFFFFF   00000004    8        00\t00\tFF\tFF\tFF\tFF\tFF\tFF\r\n      3602  1FFFFFFF   00000004    8        00\t20\tFF\tFF\tFF\tFF\tFF\tFF\r\n      3593  18F106A7   00000004    8        00\tF7\tFF\tFF\tFF\tFF\tFF\tB8\r\n      3592  1FFFFFFF   00000004    8        00\t00\tFF\tFF\tFF\tFF\tFF\tFF\r\n      3583  0CF102A7   00000004    8        30\t75\tE0\t2E\t80\tFF\tFF\tFD\r\n      3583  0CF101A7   00000004    8        68\t00\t97\tCC\t00\t19\t39\tCD\r\n      3582  1FFFFFFF   00000004    8        00\t20\tFF\tFF\tFF\tFF\tFF\tFF\r\n      3572  1FFFFFFF   00000004    8        00\t20\tFF\tFF\tFF\tFF\tFF\tFF\r\n      3563  0CF102A7   00000004    8        30\t75\tE0\t2E\t80\tFF\tFF\tFD\r\n      3563  0CF101A7   00000004    8        68\t00\t97\tCC\t00\t19\t39\tCC\r\n      3562  1FFFFFFF   00000004    8        00\t20\tFF\tFF\tFF\tFF\tFF\tFF\r\n      3552  1FFFFFFF   00000004    8        00\t00\tFF\tFF\tFF\tFF\tFF\tFF\r\n      3603  0CF101A7   00000004    8        68\t00\t97\tCC\t00\t19\t39\tCE\r\n      3602  1FFFFFFF   00000004    8        00\t20\tFF\tFF\tFF\tFF\tFF\tFF\r\n      3593  18F106A7   00000004    8        00\tF7\tFF\tFF\tFF\tFF\tFF\tB8\r\n      3592  1FFFFFFF   00000004    8        00\t00\tFF\tFF\tFF\tFF\tFF\tFF\r\n      3583  0CF102A7   00000004    8        30\t75\tE0\t2E\t80\tFF\tFF\tFD\r\n      3583  0CF101A7   00000004    8        68\t00\t97\tCC\t00\t19\t39\tCD\r\n      3582  1FFFFFFF   00000004    8        00\t20\tFF\tFF\tFF\tFF\tFF\tFF\r\n      3572  1FFFFFFF   00000004    8        00\t20\tFF\tFF\tFF\tFF\tFF\tFF\r\n      3563  0CF102A7   00000004    8        30\t75\tE0\t2E\t80\tFF\tFF\tFD\r\n      3563  0CF101A7   00000004    8        68\t00\t97\tCC\t00\t19\t39\tCC\r\n      3562  1FFFFFFF   00000004    8        00\t20\tFF\tFF\tFF\tFF\tFF\tFF\r\n      3603  0CF102A7   00000004    8        30\t75\tE0\t2E\t80\tFF\tFF\tFD\r\n      3603  0CF101A7   00000004    8        68\t00\t97\tCC\t00\t19\t39\tCE\r\n      3602  1FFFFFFF   00000004    8        00\t20\tFF\tFF\tFF\tFF\tFF\tFF\r\n      3593  18F106A7   00000004    8        00\tF7\tFF\tFF\tFF\tFF\tFF\tB8\r\n      3592  1FFFFFFF   00000004    8        00\t00\tFF\tFF\tFF\tFF\tFF\tFF\r\n      3583  0CF102A7   00000004    8        30\t75\tE0\t2E\t80\tFF\tFF\tFD\r\n      3583  0CF101A7   00000004    8        68\t00\t97\tCC\t
